vi "display FC status.vi"(7 "in or out display Refnum":refnum<vi>, 8 "error in":errorcluster={"status"=FALSE, "code"=-1950679034, "source"="Shared Variable in Large VAC READBACKS.vi<APPEND>\nThis error or warning occurred while reading the following Shared Variable:\n\\\\My Computer\\lowendshmc\\digital outputs\n\\\\192.168.1.200\\lowendshmc\\digital outputs"}, 9 "Faraday Cup Status":T1, 10 "device control Refnum":refnum<vi>, 11 "use color control":bool) -> (0 "error out":errorcluster={"status"=FALSE, "code"=-1950679034, "source"="Shared Variable in Large VAC READBACKS.vi<APPEND>\nThis error or warning occurred while reading the following Shared Variable:\n\\\\My Computer\\lowendshmc\\digital outputs\n\\\\192.168.1.200\\lowendshmc\\digital outputs"})   [LabVIEW 2016, in "sub-VIs.lvlib"]
doc: "controls the display of if a cup or apt. is in the beamline"
uses:
  sub-VIs/sub-VIs.lvlib
  controls/Faraday cup states.ctl
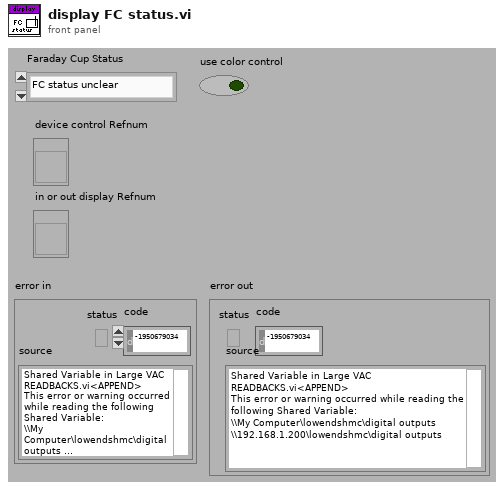
[diagram p1: front panel]
types:
  T1 = typedef "Faraday cup states.ctl" = enum16{"FC status unclear", "FC in", "FC out"}
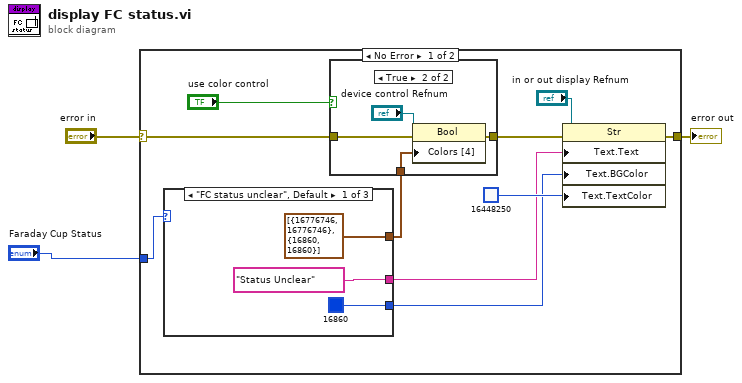
[diagram p0: block diagram]
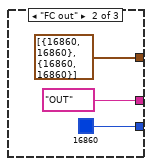
[diagram p3: hidden frame]
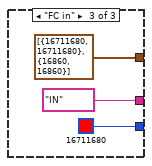
[diagram p4: hidden frame]
diagram:
  n1 = case shown="No Error" "error in" {
    selector: "error in" -> [w6 w28]
    tunnel: [w7 w28] -> w3
    tunnel: "Faraday Cup Status" -> [w4 _]
    frame No Error {
      n2 = case shown="\"FC status unclear\", Default" w4 {
        tunnel: ["Status Unclear" ("Text.Text") "OUT" ("Text.Text") "IN" ("Text.Text")] -> w10
        tunnel: [u32 16860 u32 16860 u32 16711680] -> w11
        tunnel: [cluster{u32, u32}[] [{16776746, 16776746}, {16860, 16860}] ("Colors [4]") cluster{u32, u32}[] [{16860, 16860}, {16860, 16860}] ("Colors [4]") cluster{u32, u32}[] [{16711680, 16711680}, {16860, 16860}] ("Colors [4]")] -> w13
        frame "FC status unclear", Default {
        }
        frame "FC out" {
        }
        frame "FC in" {
        }
      }
      n3 = case shown="True" "use color control" {
        tunnel: w13 -> [_ w18]
        tunnel: [w14 w17] -> w8
        tunnel: w6 -> [w14 w16]
        frame False {
        }
        frame True {
          n4 = property on="Property Node" class="Bool"(reference="device control Refnum", error in=w16, "Colors [4]"=w18) -> (error out=w17:errorcluster)  [unwired: 1 out]
        }
      }
      n5 = property on="Property Node" class="Str"(reference="in or out display Refnum", error in=w8, "Text.Text"=w10, "Text.BGColor"=w11, "Text.TextColor"=u32 16448250) -> (error out=w7:errorcluster)  [unwired: 1 out]
    }
    frame Error {
    }
  }
  "error out" <- w3
